vi "New Queue.vi"(9 "Depth":i32, 11 "Channel Data In":T1) -> (1 "Queue":refnum<queue>, 3 "Channel Data":T1)   [LabVIEW 2020, in "Flex.lvlib"]
uses:
  Flex.lvlib
  Channel Data.ctl
  Element.ctl
  Element Info.ctl
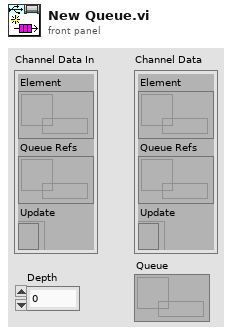
[diagram p1: front panel]
types:
  T1 = typedef "Flex.lvlib/Channel Data.ctl" = cluster{"Element":refnum<data-value>, "Queue Refs":refnum<data-value>, "Update":refnum<k4>}
  T2 = typedef "Flex.lvlib/Element.ctl" = dbl
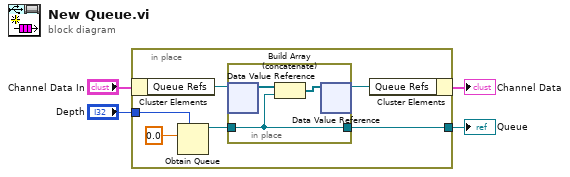
[diagram p0: block diagram]
diagram:
  n1 = in-place {
    in-place-border: "Depth" -> [w7]
    in-place-border: [w5] -> w1
    n2 = in-place-cluster #1("Channel Data In") -> ("Queue Refs"=w10:refnum<data-value>)
    n3 = Obtain Queue(max queue size (-1, unlimited)=w7, element data type=T2 0.0 ("element")) -> (queue out=w6:refnum<queue>)  [unwired: 3 in, 2 out]
    n4 = in-place {
      in-place-border: w6 -> [w11]
      in-place-border: [w11] -> w5
      n5 = in-place-dvr #2(w10) -> (w13:refnum<queue>[])  [unwired: 1 out]
      n6 = Build Array (concatenate)(w13, w11) -> (w12:refnum<queue>[])
      n7 = in-place-dvr #2(w12) -> (w9:refnum<data-value>)  [unwired: 1 out]
    }
    n8 = in-place-cluster #1("Queue Refs"=w9) -> (→"Channel Data":T1)
  }
  "Queue" <- w1
